vi "Memory.Pointer.Parameter Check.Null Pointer.vi"(7 "source vi name":string, 8 "error in (no error)":errorcluster, 11 "Pointer in":refnum<class "Memory.Pointer.lvclass">) -> (0 "error out":errorcluster, 3 "Pointer out":refnum<class "Memory.Pointer.lvclass">)   [LabVIEW 2016, in "Memory Manager.lvlib" / "Memory.Pointer.lvclass"]
uses:
  Memory.Pointer.lvclass
  Memory.Pointer.lvclass/Memory.Pointer.ctl
  Memory.Pointer.Errors.Null Pointer.vi
  Memory.Pointer.Errors.Create Error.vi
  Submodules/Static Error Handling/Source/Library/VIs/Static Error Handling.Error Cluster Constant.vi
  Submodules/Static Error Handling/Source/Library/VIs/Static Error Handling.Error Cluster Constant (256B).vi
  Submodules/Static Error Handling/Source/Library/VIs/Static Error Handling.Parameters.Status.Set.vi
  Submodules/Static Error Handling/Source/Library/VIs/Static Error Handling.Parameters.Code.Set.vi
  Submodules/Static Error Handling/Source/Library/VIs/Static Error Handling.Parameters.VI Source.Set.vi
  Constants/Memory.Constants.vi
  Constants/Memory.Constants.Library Name.vi
  Memory.Pointer.Errors.Get Info.vi
  Submodules/Static Error Handling/Source/Library/VIs/Static Error Handling.Source Buffer.Write.String.vi
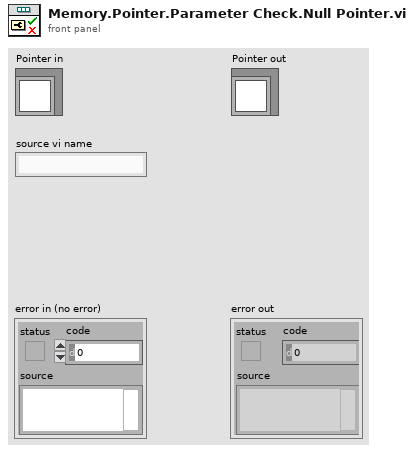
[diagram p1: front panel]
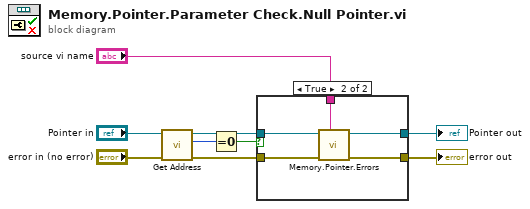
[diagram p0: block diagram]
diagram:
  n1 = call "Get Address.vi"("error in (no error)"="error in (no error)", "Pointer in"="Pointer in") -> ("error out"=w4:errorcluster, "address"=w7:u64, "Pointer out"=w2:refnum<class "Memory.Pointer.lvclass">)  [unwired: 7 in]
  n2 = Equal To 0?(x=w7) -> (x = 0?=w3:bool)
  n3 = case shown="True" w3 {
    tunnel: w2 -> [w10 w16]
    tunnel: w4 -> [w11 w14]
    tunnel: [w11 w13] -> w9
    tunnel: [w10 w15] -> w8
    tunnel: "source vi name" -> [_ w12]
    frame False {
    }
    frame True {
      n4 = call-poly "Memory.Pointer.Errors.vi"("source vi name"=w12, "error in (no error)"=w14, "pointer in"=w16) -> ("error out"=w13:errorcluster, "pointer out"=w15:refnum<class "Memory.Pointer.lvclass">)  [unwired: 7 in]
    }
  }
  "error out" <- w9
  "Pointer out" <- w8
